vi "Stop Core.vi"(10 "final error code":i32, 11 "Cli in":refnum<class "Cli.lvclass">) -> (3 "Cli out":refnum<class "Cli.lvclass">)   [LabVIEW 2022 SP3, in "Cli.lvlib" / "Cli.lvclass"]
doc: "(<B>Filename</B>: Actor Framework.lvlib:Actor.lvclass:Stop Core.vi)\n\nDefines what the actor does before it stops. Use the <B>final error code</B> input to determine whether the actor shut down in response to an error.\n\nBy default, this method does nothing. A descendant class may override it to define behavior, such as shutting down any processes the actor initiated in its override of the Actor Core method."
uses:
  Cli.lvclass
  Cli.lvclass/Cli.ctl
  <vilib>/ActorFramework/Actor/Actor.lvclass
  ArgumentParser/Source/ArgumentParser/ArgumentParser.lvclass
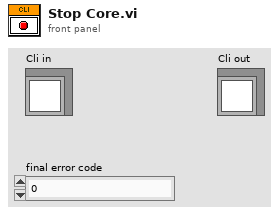
[diagram p1: front panel]
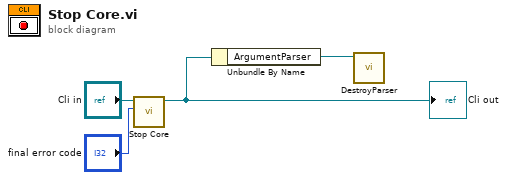
[diagram p0: block diagram]
diagram:
  n1 = call-parent "Stop Core.vi"("final error code"="final error code", "Actor in"="Cli in") -> ("Actor out"=w2:refnum<class "Cli.lvclass">)  [unwired: 9 in]
  "Cli out" <- w2
  n2 = Unbundle By Name(w2) -> ("ArgumentParser"=w1:refnum<class "ArgumentParser.lvclass">)
  n3 = call-dynamic "DestroyParser.vi"("ArgumentParser in"=w1) -> ()  [unwired: 10 in, 1 out]
